vi "multimeter.vi"() -> ()   [LabVIEW 2018]
panel:
  out "Numeric":i32
  out "RMS":dbl
  in  "stop":bool
  out "Waveform Chart":dbl(graph)
  out "value":dbl
  in  "function (Vdc:1)":u16(ring)=1 items=["ac voltage", "dc voltage", "2-wire resistance", "4-wire resistance", "ac current", "dc current", "frequency", "temperature"]
  out "Reading Result":string
  out "error out":T1
  in  "error in":T1
  in  "GPIB Address":string="16"
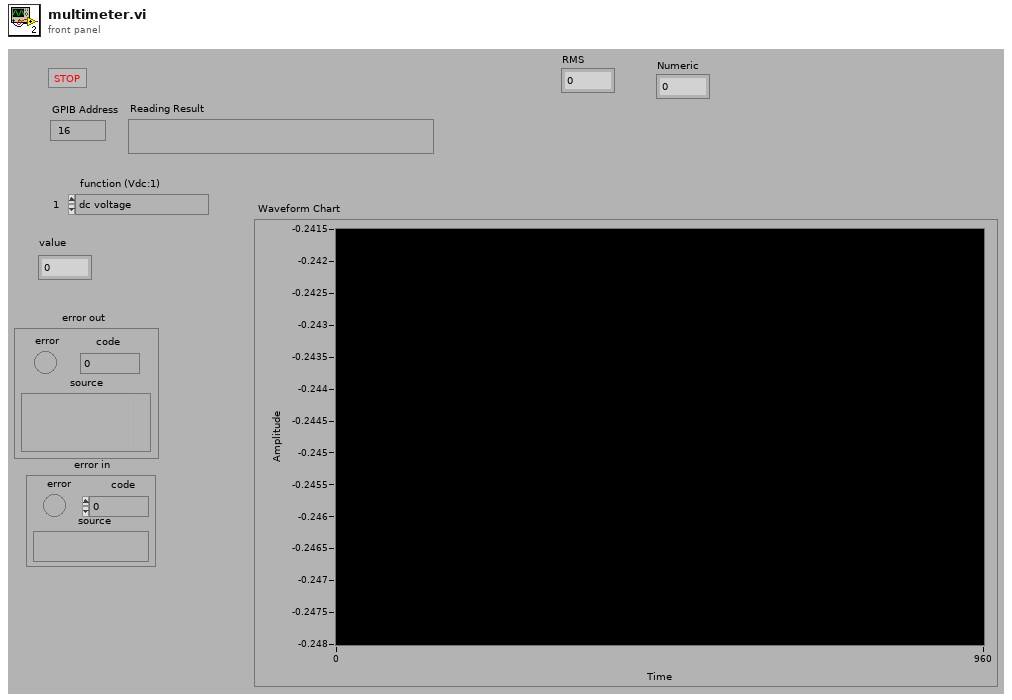
[diagram p1: front panel]
types:
  T1 = cluster{"error":bool, "code":i32, "source":string}
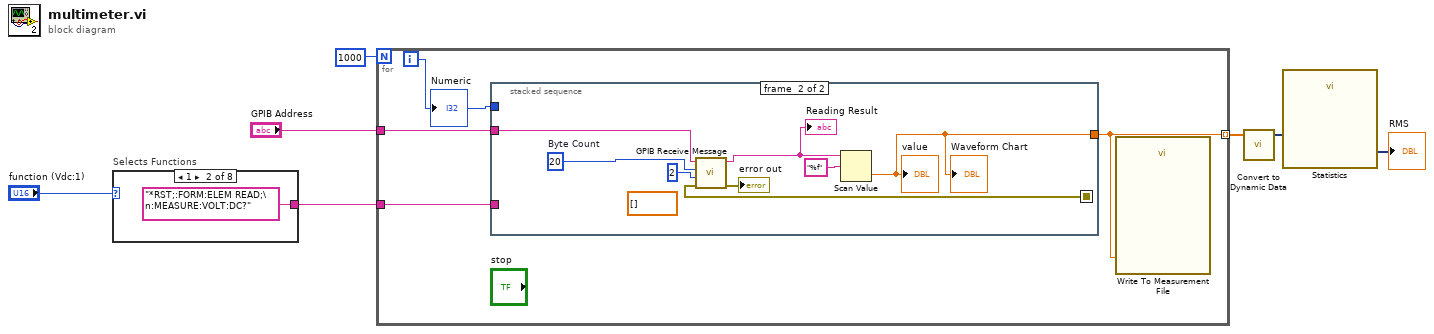
[diagram p0: block diagram]
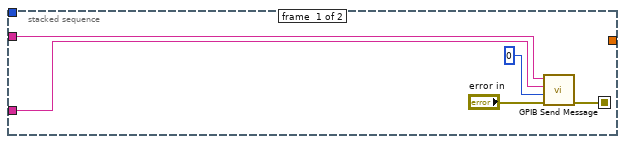
[diagram p2: hidden frame]
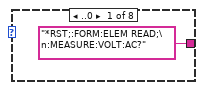
[diagram p3: hidden frame]
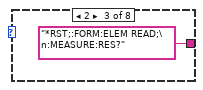
[diagram p4: hidden frame]
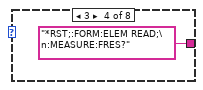
[diagram p5: hidden frame]
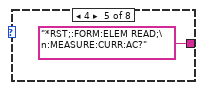
[diagram p6: hidden frame]
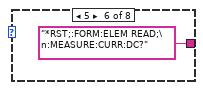
[diagram p7: hidden frame]
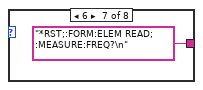
[diagram p8: hidden frame]
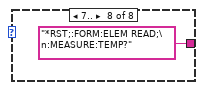
[diagram p9: hidden frame]
diagram:
  n1 = case "Selects Functions" shown="1" "function (Vdc:1)" {
    tunnel: ["*RST;:FORM:ELEM READ;\n:MEASURE:VOLT:AC?" "*RST;:FORM:ELEM READ;\n:MEASURE:VOLT:DC?" "*RST;:FORM:ELEM READ;\n:MEASURE:RES?" "*RST;:FORM:ELEM READ;\n:MEASURE:FRES?" "*RST;:FORM:ELEM READ;\n:MEASURE:CURR:AC?" "*RST;:FORM:ELEM READ;\n:MEASURE:CURR:DC?" "*RST;:FORM:ELEM READ; :MEASURE:FREQ?\n" "*RST;:FORM:ELEM READ;\n:MEASURE:TEMP?"] -> w5
    frame ..0 {
    }
    frame 1 {
    }
    frame 2 {
    }
    frame 3 {
    }
    frame 4 {
    }
    frame 5 {
    }
    frame 6 {
    }
    frame 7.. {
    }
  }
  n2 = for {
    N: 1000 -> [_]
    tunnel: "GPIB Address" -> [w19]
    tunnel: w5 -> [w18]
    tunnel: [w16] -> w2 mode=indexing
    i -> [w17]
    n3 = stacked-sequence {
      seq-local: [w20 _] -> [_ w29]
      tunnel: w19 -> [w24 w32]
      tunnel: w18 -> [w21 _]
      tunnel: w17 -> [_ _]
      tunnel: [_ w25] -> w16
      frame #0 {
        n4 = call "GPIB Send Message.vi"("address string"=w24, "write buffer"=w21, "write mode (set END:0)"=0, "error in"="error in") -> ("error out"=w20:T1)  [unwired: 3 in, 2 out]
      }
      frame #1 {
        (unwired) dbl[] [] ("Waveform Graph")
        w31 = 20  # Byte Count
        n5 = call "GPIB Receive Message.vi"("address string"=w32, "byte count"=w31, "read mode"=2, "error in"=w29) -> ("read buffer"=w27:string, "error out"=→"error out":T1)  [unwired: 3 in, 1 out]
        "Reading Result" <- w27
        n6 = Scan Value(string=w27, format string="%f") -> (value=w25:dbl)  [unwired: 1 in, 1 out]
        "value" <- w25
        "Waveform Chart" <- w25
      }
    }
    n7 = call "Write To Measurement File"("Signals"=w16) -> ()  [unwired: 16 in, 3 out]
    "Numeric" <- w17
  }
  n8 = call "Convert to Dynamic Data"("Array"=w2) -> ("Dynamic Data Type"=w1:dynamicdata)  [unwired: 3 in]
  n9 = call "Statistics"("Signals"=w1) -> ("RMS"=→"RMS":dynamicdata)  [unwired: 25 in, 1 out]
